vi "Hybrid User Control.vi"(2 "error out":errorcluster, 3 "Old User Control":bool, 4 "User Control":bool, 5 "VI Refnum":refnum<vi>) -> (0 "error out 2":errorcluster, 1 "dup VI Refnum":refnum<vi>)   [LabVIEW 2024]
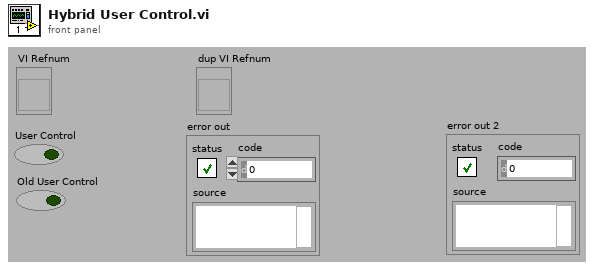
[diagram p1: front panel]
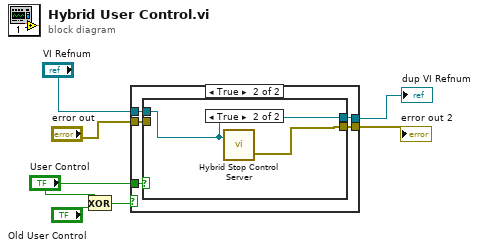
[diagram p0: block diagram]
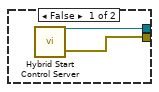
[diagram p3: hidden frame]
diagram:
  n1 = Exclusive Or(1:"Old User Control", 2:"User Control") -> (0:w5:bool)
  n2 = case shown="True" w5 {
    tunnel: [w9 w14] -> w1
    tunnel: [w8 w13] -> w2
    tunnel: "VI Refnum" -> [w8 w10]
    tunnel: "error out" -> [w9 w12]
    tunnel: "User Control" -> [_ w11]
    frame False {
    }
    frame True {
      n3 = case shown="True" w11 {
        tunnel: w10 -> [_ w18]
        tunnel: w12 -> [_ _]
        tunnel: [w16 w18] -> w13
        tunnel: [w15 w17] -> w14
        frame False {
          n4 = call "Hybrid Start Control Server.vi"() -> ("error out"=w15:errorcluster, "dup reference"=w16:refnum<vi>)
        }
        frame True {
          n5 = call "Hybrid Stop Control Server.vi"("dup reference"=w18) -> ("error out"=w17:errorcluster)  [unwired: 2 in]
        }
      }
    }
  }
  "dup VI Refnum" <- w2
  "error out 2" <- w1
